vi "Calculate Movement Ratios.vi"(2 "error in (no error)":errorcluster, 3 "Car.lvclass":refnum<class "Car.lvclass">) -> (0 "error out":errorcluster, 1 "Car.lvclass 2":refnum<class "Car.lvclass">)   [LabVIEW 2015, in "Car.lvclass"]
uses:
  Car.lvclass
  Car.lvclass/Car.ctl
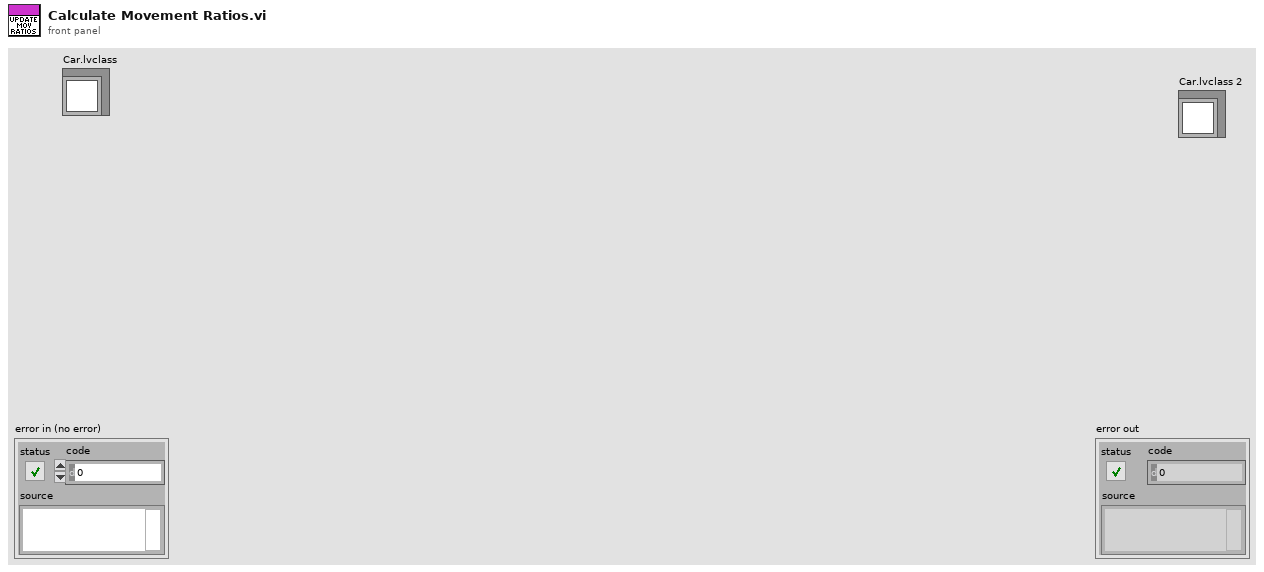
[diagram p1: front panel]
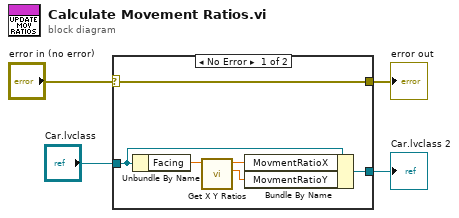
[diagram p0: block diagram]
diagram:
  n1 = case shown="No Error" "error in (no error)" {
    selector: "error in (no error)" -> [w10 w12]
    tunnel: [w10 w12] -> w3
    tunnel: [w8 w11] -> w2
    tunnel: "Car.lvclass" -> [w9 w11]
    frame No Error {
      n2 = Unbundle By Name(w9) -> ("Facing"=w7:dbl)
      n3 = call "Get X Y Ratios.vi"("Facing"=w7) -> ("Y Ratio"=w6:dbl, "X Ratio"=w5:dbl)  [unwired: 9 in]
      n4 = Bundle By Name(cluster=w9, "MovmentRatioX"=w5, "MovmentRatioY"=w6) -> (w8:refnum<class "Car.lvclass">)
    }
    frame Error {
    }
  }
  "Car.lvclass 2" <- w2
  "error out" <- w3
